vi "Drive Train Update Metrics.vi"(10 "Input":T1) -> (2 "Output":T1)   [LabVIEW 2013]
uses:
  Drive Train Metrics.ctl
  CmdFlag.ctl
panel:
  out "Right Distance":dbl(graph)
  out "Left Distance":dbl(graph)
  out "Right Rate":dbl(graph)
  out "Left Rate":dbl(graph)
  out "Acceleration":dbl(graph)
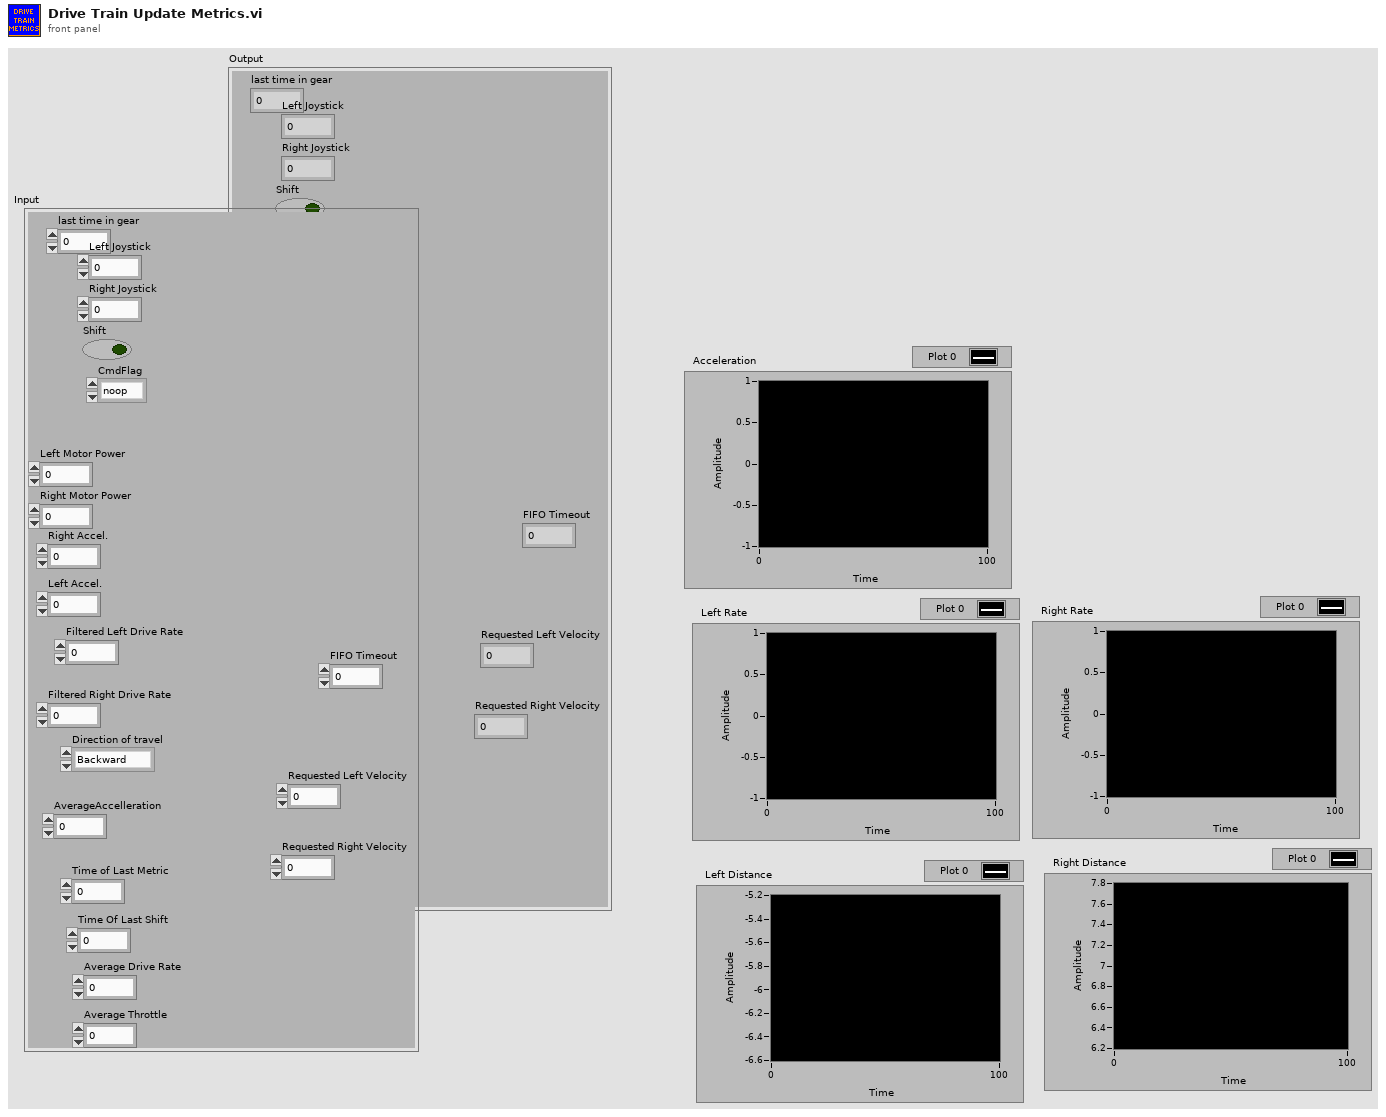
[diagram p1: front panel]
types:
  T1 = typedef "Drive Train Metrics.ctl" = cluster{"last time in gear":u32, "Shift":bool, "Right Joystick":dbl, "Left Joystick":dbl, "CmdFlag":T2, "Right Motor Power":dbl, "Left Motor Power":dbl, "Right Accel.":dbl, "Left Accel.":dbl, "Filtered Left Drive Rate":dbl, "Filtered Right Drive Rate":dbl, "Direction of travel":enum16{"Backward", "Forward", "Spin"}, "AverageAccelleration":dbl, "Time of Last Metric":u32, "Time Of Last Shift":dbl, "Average Drive Rate":dbl, "Average Throttle":dbl, "FIFO Timeout":i32, "Requested Left Velocity":dbl, "Requested Right Velocity":dbl}
  T2 = typedef "CmdFlag.ctl" = enum16{"noop", "suspend", "resume"}
  T3 = typedef "WPI_EncoderDevRef.ctl" = cluster{"DevStatus":errorcluster, "EncoderIndex":T4, "CounterIndex":T5, "DistancePerCount":dbl, "Decoding Type":T6}
  T4 = typedef "FPGA_EncoderIdx.ctl" = enum8{"Enc 0", "Enc 1", "Enc 2", "Enc 3", "Invalid"}
  T5 = typedef "FPGA_CounterCtrSystemIndex.ctl" = enum8{"Ctr 0", "Ctr 1", "Ctr 2", "Ctr 3", "Ctr 4", "Ctr 5", "Ctr 6", "Ctr 7", "Invalid"}
  T6 = typedef "WPI_EncoderType.ctl" = enum16{"1x", "2x", "4x"}
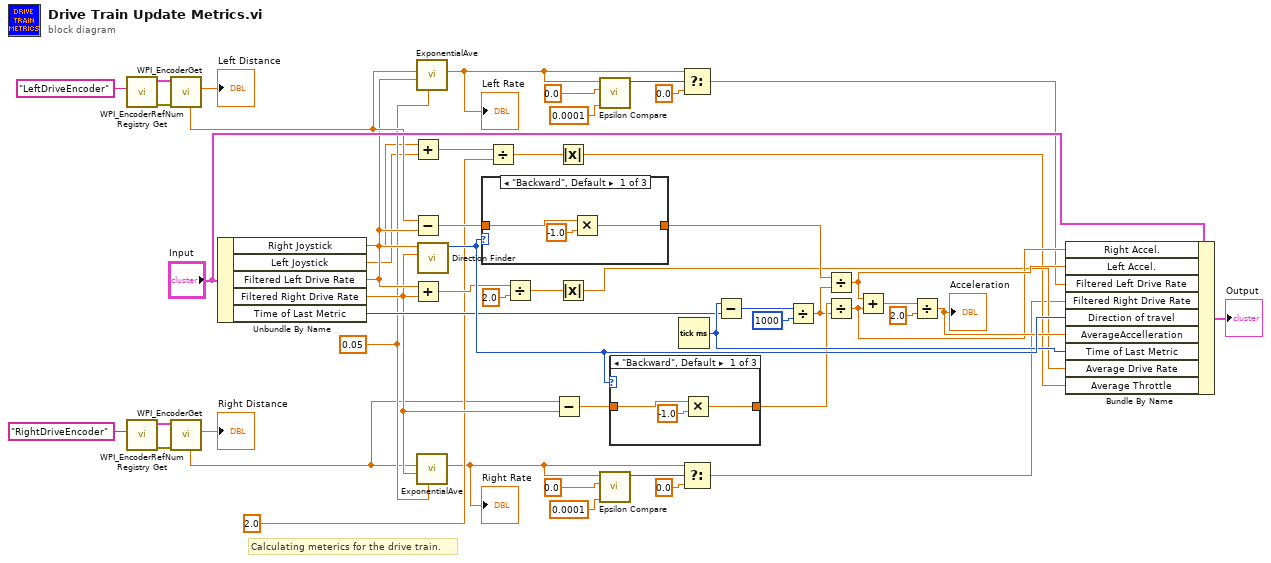
[diagram p0: block diagram]
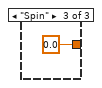
[diagram p3: hidden frame]
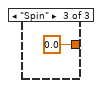
[diagram p5: hidden frame]
diagram:
  w20 = 0.05 ("Coff")
  # "Calculating meterics for the drive train."
  n1 = call <vilib>:"WPI_EncoderRefNum Registry Get.vi"("refnum name"="LeftDriveEncoder") -> ("error out"=w51:errorcluster, "EncoderDevRef"=w50:T3)  [unwired: 9 in]
  n2 = call <vilib>:"WPI_EncoderRefNum Registry Get.vi"("refnum name"="RightDriveEncoder") -> ("error out"=w48:errorcluster, "EncoderDevRef"=w47:T3)  [unwired: 9 in]
  n3 = call <vilib>:"WPI_EncoderGet.vi"("error in (no error)"=w51, "EncoderDevRef"=w50) -> ("Distance"=→"Left Distance":dbl, "Rate"=w31:dbl)  [unwired: 4 in, 4 out]
  n4 = call <vilib>:"WPI_EncoderGet.vi"("error in (no error)"=w48, "EncoderDevRef"=w47) -> ("Distance"=→"Right Distance":dbl, "Rate"=w1:dbl)  [unwired: 4 in, 4 out]
  n5 = Unbundle By Name("Input") -> ("Right Joystick"=w15:dbl, "Left Joystick"=w14:dbl, "Filtered Left Drive Rate"=w26:dbl, "Filtered Right Drive Rate"=w25:dbl, "Time of Last Metric"=w37:u32)
  n6 = Add(x=w15, y=w14) -> (x+y=w19:dbl)
  n7 = Subtract(x=w31, y=w26) -> (x-y=w42:dbl)
  n8 = Add(x=w26, y=w25) -> (x+y=w27:dbl)
  n9 = call "ExponentialAve.vi"("Coff"=w20, "PreviousValue"=w26, "InputValue"=w31) -> ("Smoothed Value"=w10:dbl)  [unwired: 8 in]
  "Left Rate" <- w10
  n10 = call "ExponentialAve.vi"("Coff"=w20, "PreviousValue"=w25, "InputValue"=w1) -> ("Smoothed Value"=w3:dbl)  [unwired: 8 in]
  "Right Rate" <- w3
  n11 = call "Direction Finder.vi"("Filtered Right Drive Rate"=w25, "Filtered Left Drive Rate"=w26) -> ("Direction of travel"=w43:enum16{"Backward", "Forward", "Spin"})  [unwired: 9 in]
  n12 = case shown="\"Backward\", Default" w43 {
    tunnel: [w53 w56 0.0] -> w35
    tunnel: w42 -> [w54 w56 _]
    frame "Backward", Default {
      n13 = Multiply(x=w54, y=-1.0) -> (x*y=w53:dbl)
    }
    frame "Forward" {
    }
    frame "Spin" {
    }
  }
  n14 = Divide(x=w19, y=2.0) -> (x/y=w17:dbl)
  n15 = Divide(x=w27, y=2.0) -> (x/y=w24:dbl)
  n16 = Subtract(x=w1, y=w25) -> (x-y=w44:dbl)
  n17 = Absolute Value(x=w17) -> (abs(x)=w16:dbl)
  n18 = Absolute Value(x=w24) -> (abs(x)=w23:dbl)
  n19 = call "Epsilon Compare.vi"("Epsilon"=0.0001, "Value2"=0.0, "Value1"=w10) -> ("Boolean"=w11:bool)  [unwired: 8 in]
  n20 = call "Epsilon Compare.vi"("Epsilon"=0.0001, "Value2"=0.0, "Value1"=w3) -> ("Boolean"=w5:bool)  [unwired: 8 in]
  n21 = case shown="\"Backward\", Default" w43 {
    tunnel: [w58 w61 0.0] -> w36
    tunnel: w44 -> [w59 w61 _]
    frame "Backward", Default {
      n22 = Multiply(x=w59, y=-1.0) -> (x*y=w58:dbl)
    }
    frame "Forward" {
    }
    frame "Spin" {
    }
  }
  n23 = Tick Count (ms)() -> (millisecond timer value=w38:u32)
  n24 = Select(t=w10, s=w11, f=0.0) -> (s? t:f=w8:dbl)
  n25 = Select(t=w3, s=w5, f=0.0) -> (s? t:f=w2:dbl)
  n26 = Subtract(x=w38, y=w37) -> (x-y=w34:u32)
  n27 = Divide(x=w34, y=u32 1000) -> (x/y=w22:dbl)
  n28 = Divide(x=w35, y=w22) -> (x/y=w33:dbl)
  n29 = Divide(x=w36, y=w22) -> (x/y=w32:dbl)
  n30 = Add(x=w33, y=w32) -> (x+y=w41:dbl)
  n31 = Divide(x=w41, y=2.0) -> (x/y=w39:dbl)
  "Acceleration" <- w39
  n32 = Bundle By Name(cluster="Input", "Right Accel."=w32, "Left Accel."=w33, "Filtered Left Drive Rate"=w8, "Filtered Right Drive Rate"=w2, "Direction of travel"=w43, "AverageAccelleration"=w39, "Time of Last Metric"=w38, "Average Drive Rate"=w23, "Average Throttle"=w16) -> (→"Output":T1)
